vi "fpga_select_channel.vi"(10 "sgl 8ch":T1, 11 "channel":T2) -> (3 "value":sgl)   [LabVIEW 2021]
doc: "Get a value of specified channel."
uses:
  fpga_dtype_channel.ctl
  fpga_dtype_sgl_8ch.ctl
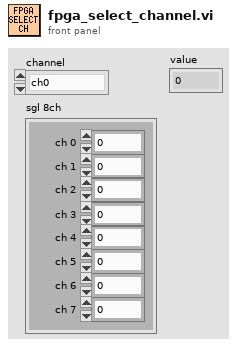
[diagram p1: front panel]
types:
  T1 = typedef "fpga_dtype_sgl_8ch.ctl" = cluster{"ch 0":sgl, "ch 1":sgl, "ch 2":sgl, "ch 3":sgl, "ch 4":sgl, "ch 5":sgl, "ch 6":sgl, "ch 7":sgl}
  T2 = typedef "fpga_dtype_channel.ctl" = enum16{"ch0", "ch1", "ch2", "ch3", "ch4", "ch5", "ch6", "ch7"}
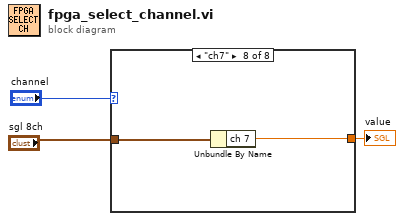
[diagram p0: block diagram]
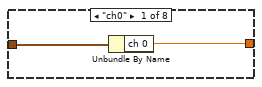
[diagram p2: hidden frame]
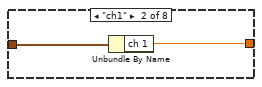
[diagram p3: hidden frame]
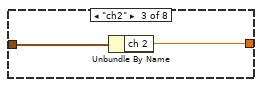
[diagram p4: hidden frame]
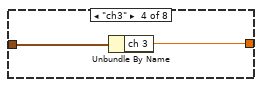
[diagram p5: hidden frame]
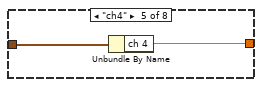
[diagram p6: hidden frame]
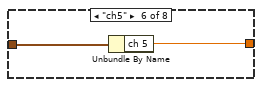
[diagram p7: hidden frame]
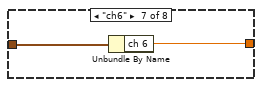
[diagram p8: hidden frame]
diagram:
  n1 = case shown="\"ch7\"" "channel" {
    tunnel: "sgl 8ch" -> [w5 w7 w9 w11 w13 w15 w17 w19]
    tunnel: [w4 w6 w8 w10 w12 w14 w16 w18] -> w1
    frame "ch0" {
      n2 = Unbundle By Name(w5) -> ("ch 0"=w4:sgl)
    }
    frame "ch1" {
      n3 = Unbundle By Name(w7) -> ("ch 1"=w6:sgl)
    }
    frame "ch2" {
      n4 = Unbundle By Name(w9) -> ("ch 2"=w8:sgl)
    }
    frame "ch3" {
      n5 = Unbundle By Name(w11) -> ("ch 3"=w10:sgl)
    }
    frame "ch4" {
      n6 = Unbundle By Name(w13) -> ("ch 4"=w12:sgl)
    }
    frame "ch5" {
      n7 = Unbundle By Name(w15) -> ("ch 5"=w14:sgl)
    }
    frame "ch6" {
      n8 = Unbundle By Name(w17) -> ("ch 6"=w16:sgl)
    }
    frame "ch7" {
      n9 = Unbundle By Name(w19) -> ("ch 7"=w18:sgl)
    }
  }
  "value" <- w1
